vi "Create Response Headers.vi"(5 "Response Headers in":refnum<class "Response Headers.lvclass">, 8 "error in (no error)":errorcluster, 11 "Response Headers":string) -> (0 "error out":errorcluster, 3 "Response Headers out":refnum<class "Response Headers.lvclass">)   [LabVIEW 2020, in "REST Client.lvlib" / "Response Headers.lvclass"]
uses:
  Response Headers.lvclass
  Response Headers.lvclass/Response Headers.ctl
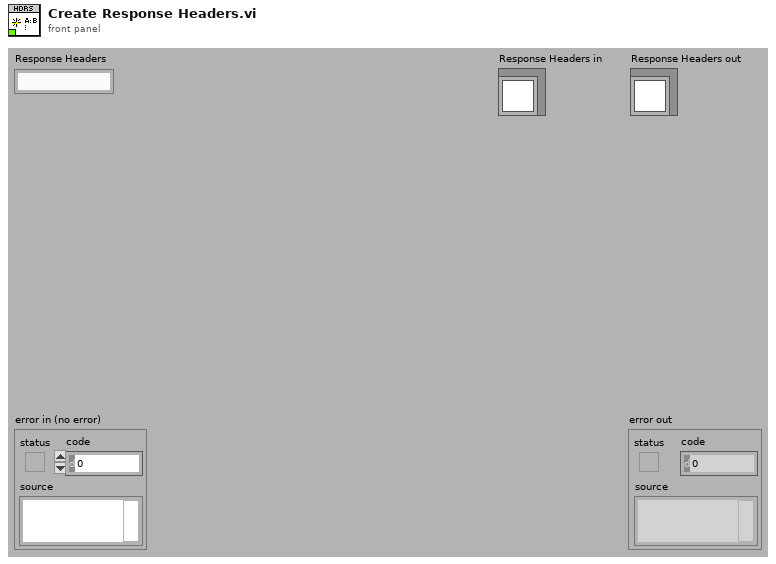
[diagram p1: front panel]
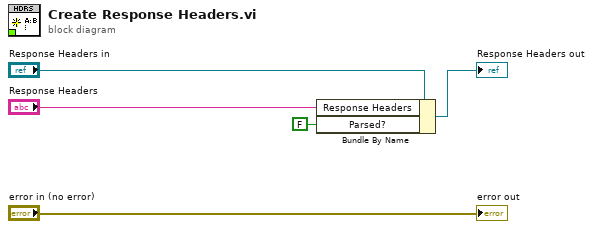
[diagram p0: block diagram]
diagram:
  n1 = Bundle By Name(cluster="Response Headers in", "Response Headers"="Response Headers", "Parsed?"=FALSE) -> (→"Response Headers out":refnum<class "Response Headers.lvclass">)
  "error out" <- "error in (no error)"
